vi "Time String(s).vi"() -> (2 "system time string(s)":string)   [LabVIEW 2020]
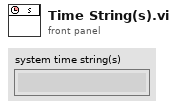
[diagram p1: front panel]
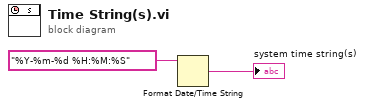
[diagram p0: block diagram]
diagram:
  n1 = Format Date/Time String(time format string (%c)="%Y-%m-%d %H:%M:%S") -> (date/time string=→"system time string(s)":string)  [unwired: 2 in]
